vi "Read IP Address of Server.vi"(8 "error in (no error)":errorcluster, 11 "Client Config in":refnum<class "Client Config.lvclass">) -> (0 "error out":errorcluster, 2 "IP Address of Server":string, 3 "Client Config out":refnum<class "Client Config.lvclass">)   [LabVIEW 2026, in "Client Controller.lvlib" / "Client Config.lvclass"]
uses:
  Client Config.lvclass
  Client Config.lvclass/Client Config.ctl
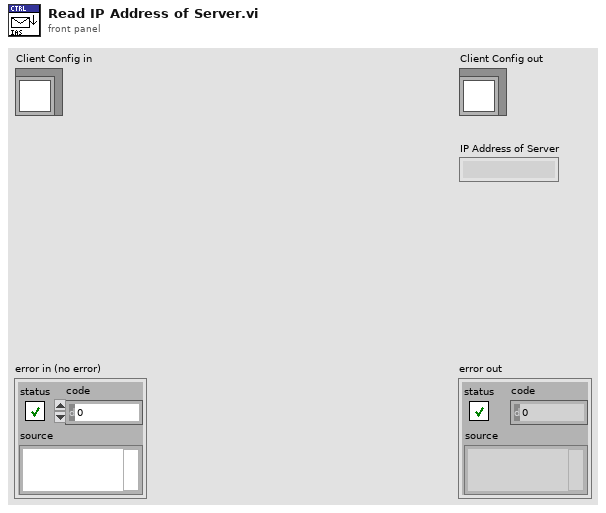
[diagram p1: front panel]
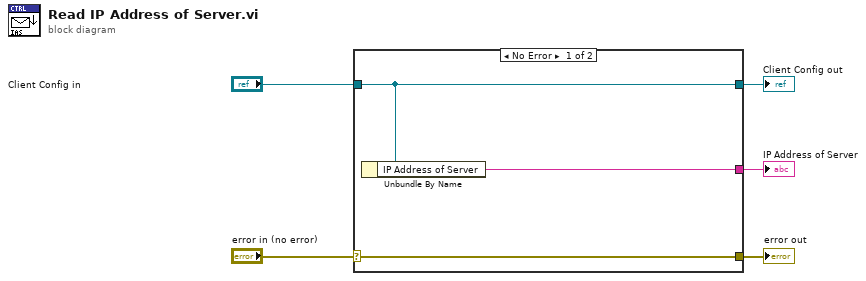
[diagram p0: block diagram]
diagram:
  n1 = case shown="No Error" "error in (no error)" {
    selector: "error in (no error)" -> [w8 w9]
    tunnel: [w8 w9] -> w4
    tunnel: [w7 w10] -> w2
    tunnel: "Client Config in" -> [w7 w10]
    tunnel: [w6 _] -> w1
    frame No Error {
      n2 = Unbundle By Name(w7) -> ("IP Address of Server"=w6:string)
    }
    frame Error {
    }
  }
  "error out" <- w4
  "Client Config out" <- w2
  "IP Address of Server" <- w1
